vi "WPI_MotorControlGetOutput.vi"(8 "error in":errorcluster, 11 "MotorControlDevRef":T1={"DeviceStatus"={"status"=FALSE, "code"=0, "source"=""}, "Type"=enum."PWM", "PWM"={"PWM Channel"=enum."Invalid", "DeadBand"={"Name"="", "maxPositivePwm"=0, "minPositivePwm"=0, "centerPwm"=0, "maxNegativePwm"=0, "minNegativePwm"=0, "angularRange"=0}}, "CAN"={"Device Number"=0, "SetOutput VI Ref"=variant(refnum<vi> refnum), "GetOutput VI Ref"=variant(refnum<vi> refnum), "Enable VI Ref"=variant(refnum<vi> refnum), "Disable VI Ref"=variant(refnum<vi> refnum), "Data"=variant}, "Invert"=FALSE, "DIO PWM"={"PWM \"Enable\" Channel"=enum."Invalid", "DIOChannel"=enum."Invalid", "PWM Rate"=0.0}}) -> (0 "error out":errorcluster, 2 "Output":dbl, 3 "MotorControlDevRef":T1={"DeviceStatus"={"status"=FALSE, "code"=0, "source"=""}, "Type"=enum."PWM", "PWM"={"PWM Channel"=enum."Invalid", "DeadBand"={"Name"="", "maxPositivePwm"=0, "minPositivePwm"=0, "centerPwm"=0, "maxNegativePwm"=0, "minNegativePwm"=0, "angularRange"=0}}, "CAN"={"Device Number"=0, "SetOutput VI Ref"=variant(refnum<vi> refnum), "GetOutput VI Ref"=variant(refnum<vi> refnum), "Enable VI Ref"=variant(refnum<vi> refnum), "Disable VI Ref"=variant(refnum<vi> refnum), "Data"=variant}, "Invert"=FALSE, "DIO PWM"={"PWM \"Enable\" Channel"=enum."Invalid", "DIOChannel"=enum."Invalid", "PWM Rate"=0.0}})   [LabVIEW 2025]
doc: "Returns the last output value or set-point that was written to the motor controller with the <B>Set Output</B> VI."
uses:
  <vilib>/Rock Robotics/WPI/MotorControl/WPI_MotorControlDeviceRef.ctl
  <vilib>/Rock Robotics/WPI/MotorControl/WPI_MotorControlType.ctl
  <vilib>/Rock Robotics/SystemInterfaces/DIO/FPGA_DIOPWMChannel.ctl
  <vilib>/Rock Robotics/WPI/PWM/WPI_PWMDeadband.ctl
  <vilib>/Rock Robotics/SystemInterfaces/DIO/FPGA_DIOChannel.ctl
  <vilib>/Rock Robotics/WPI/PWM/WPI_PWMChannelCacheOp.ctl
  <vilib>/Rock Robotics/WPI/MotorControl/WPI_MotorControlGetOutputRefType.ctl
  <vilib>/Rock Robotics/WPI/DigitalOutput/WPI_DigitalOutputDevRef.ctl
  <vilib>/Rock Robotics/WPI/Simulation/Protocol/Devices/PWM/PWM Update Ops.ctl
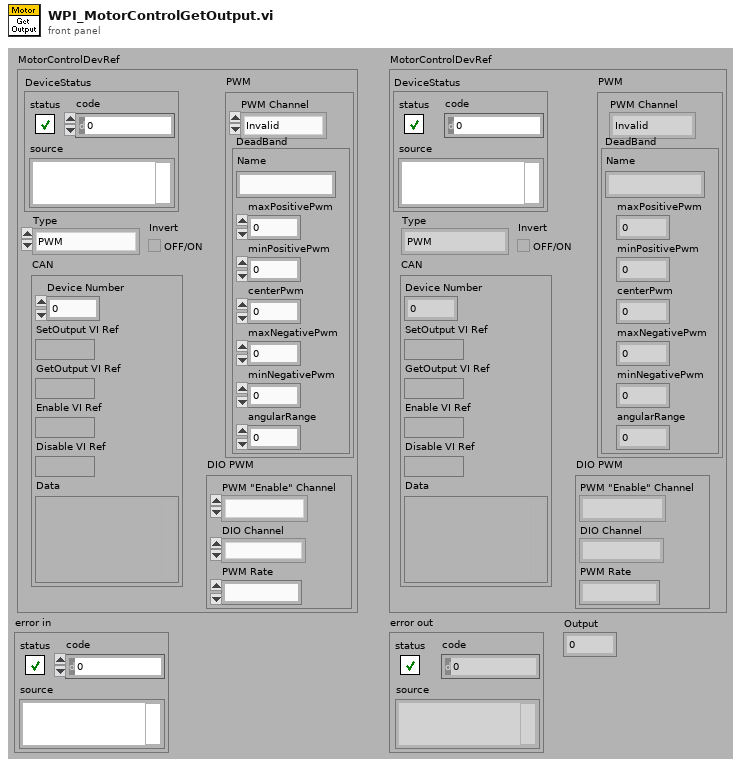
[diagram p1: front panel]
types:
  T1 = typedef "WPI_MotorControlDeviceRef.ctl" = cluster{"DeviceStatus":errorcluster, "Type":T2, "PWM":cluster{"PWM Channel":T3, "DeadBand":T4}, "CAN":cluster{"Device Number":u8, "SetOutput VI Ref":variant, "GetOutput VI Ref":variant, "Enable VI Ref":variant, "Disable VI Ref":variant, "Data":variant}, "Invert":bool, "DIO PWM":cluster{"PWM \"Enable\" Channel":T3, "DIOChannel":T5, "PWM Rate":dbl}}
  T2 = typedef "WPI_MotorControlType.ctl" = enum16{"PWM", "CAN", "DIO PWM"}
  T3 = typedef "FPGA_DIOPWMChannel.ctl" = enum8{"PWM 0", "PWM 1", "PWM 2", "PWM 3", "PWM 4", "PWM 5", "PWM 6", "PWM 7", "PWM 8", "PWM 9", "PWM MXP 0", "PWM MXP 1", "PWM MXP 2", "PWM MXP 3", "PWM MXP 4", "PWM MXP 5", "PWM MXP 6", "PWM MXP 7", "PWM MXP 8", "PWM MXP 9", "Invalid"}
  T4 = typedef "WPI_PWMDeadband.ctl" = cluster{"Name":string, "maxPositivePwm":i32, "minPositivePwm":i32, "centerPwm":i32, "maxNegativePwm":i32, "minNegativePwm":i32, "angularRange":u16}
  T5 = typedef "FPGA_DIOChannel.ctl" = enum8{"DIO 0", "DIO 1", "DIO 2", "DIO 3", "DIO 4", "DIO 5", "DIO 6", "DIO 7", "DIO 8", "DIO 9", "DIO MXP 0", "DIO MXP 1", "DIO MXP 2", "DIO MXP 3", "DIO MXP 4", "DIO MXP 5", "DIO MXP 6", "DIO MXP 7", "DIO MXP 8", "DIO MXP 9", "DIO MXP 10", "DIO MXP 11", "DIO MXP 12", "DIO MXP 13", "DIO MXP 14", "DIO MXP 15", "SPI Port CS1", "SPI Port CS2", "SPI Port CS3", "SPI Port MISO", "SPI Port MOSI", "Invalid"}
  T6 = typedef "WPI_MotorControlGetOutputRefType.ctl" = refnum<vi>
  T7 = typedef "WPI_DigitalOutputDevRef.ctl" = cluster{"DIO Channel":T5, "DevStatus":errorcluster}
  T8 = typedef "PWM Update Ops.ctl" = enum16{"set init", "set speed", "set position", "set raw", "set  period_scale", "set zero_latch", "set angular range", "get", "delete", "JSON update", "set name", "transmit initial", "reset"}
  T9 = typedef "WPI_PWMChannelCacheOp.ctl" = enum16{"Acquire", "Release", "Status"}
  T10 = typedef "WPI_PWMDeviceRef.ctl" = cluster{"DeviceStatus":errorcluster, "PWM Channel":T3}
  T11 = typedef "PWM proto.ctl" = cluster{"type":string, "device":string, "name":string, "data":T12}
  T12 = typedef "PWM data proto.ctl" = cluster{"<init":bool, "<speed":dbl, "<position":dbl, "<raw":dbl, "<period_scale":dbl, "<zero_latch":bool, "<servo range":dbl}
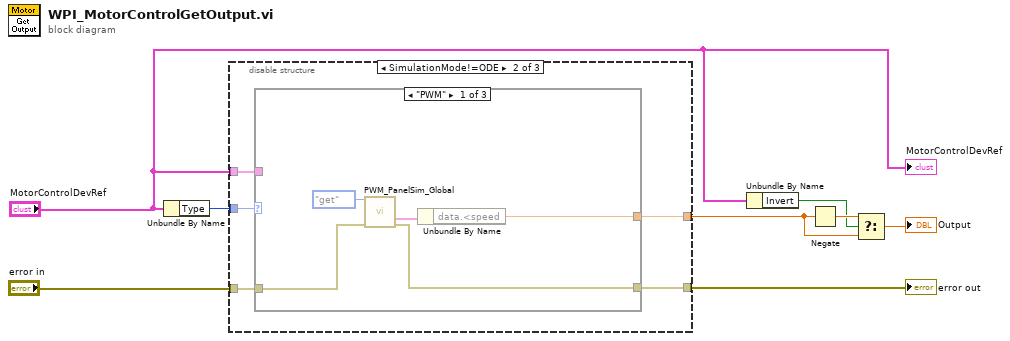
[diagram p0: block diagram]
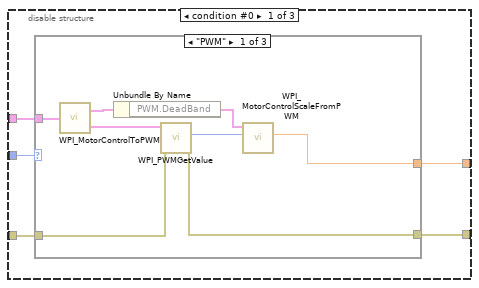
[diagram p2: hidden frame]
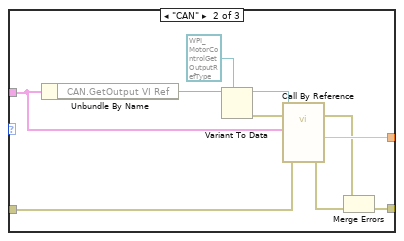
[diagram p3: hidden frame]
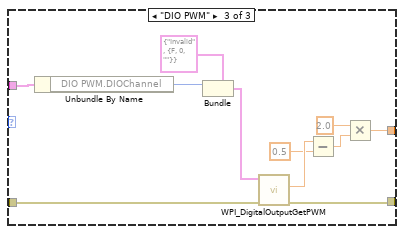
[diagram p4: hidden frame]
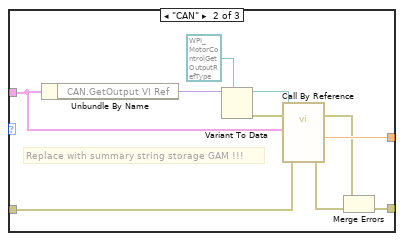
[diagram p5: hidden frame]
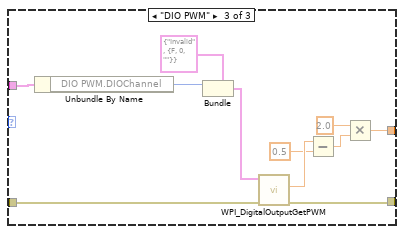
[diagram p6: hidden frame]
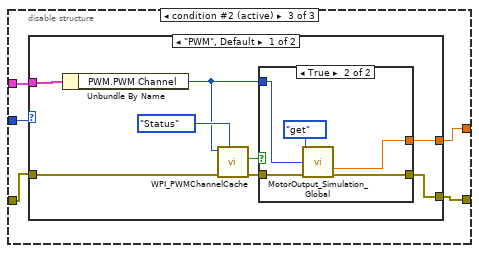
[diagram p7: hidden frame]
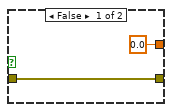
[diagram p8: hidden frame]
diagram:
  n1 = Unbundle By Name("MotorControlDevRef") -> ("Type"=w2:T2)
  n2 = disable-structure shown="SimulationMode!=ODE" {
    disable-tunnel: "error in" -> [w13 w45 w76]
    disable-tunnel: "MotorControlDevRef" -> [w12 w43 w78]
    disable-tunnel: [w11 w47 w74] -> w6
    disable-tunnel: w2 -> [w10 w44 w77]
    disable-tunnel: [w9 w46 w75] -> w1
    frame condition #0 {
      n3 = case shown="\"PWM\"" w10 {
        tunnel: [w14 w23 w37] -> w11
        tunnel: w12 -> [w17 w27 w42]
        tunnel: w13 -> [w15 w29 w38]
        tunnel: [w20 w30 w33] -> w9
        frame "PWM" {
          n4 = call <vilib>:"WPI_MotorControlToPWM.vi"("MotorControlDeviceRef"=w17) -> ("MotorControlDeviceRef"=w16:T1, "PWMDeviceRef"=w19:T10)
          n5 = Unbundle By Name(w16) -> ("PWM.DeadBand"=w18:T4)
          n6 = call <vilib>:"WPI_PWMGetValue.vi"("error in (no error)"=w15, "PWMDeviceRef"=w19) -> ("error out"=w14:errorcluster, "Value"=w21:u16)  [unwired: 8 out]
          n7 = call <vilib>:"WPI_MotorControlScaleFromPWM.vi"("Raw PWM Value"=w21, "DeadBand Info"=w18) -> ("Output (1,-1)"=w20:dbl)  [unwired: 9 out]
        }
        frame "CAN" {
          n8 = Unbundle By Name(w27) -> ("CAN.GetOutput VI Ref"=w31:variant)
          n9 = Variant To Data(type=T6 refnum ("MotorControlGetOutput"), Variant=w31) -> (data=w28:T6, error out=w26:errorcluster)  [unwired: 1 in]
          n10 = call-by-ref "?"(reference=w28, error in=w26, "error in"=w29, "MotorControlDevRef"=w27) -> (error out=w25:errorcluster, 0:"error out"=w24:errorcluster, "Output"=w30:dbl)  [unwired: 7 in, 2 out]
          n11 = Merge Errors(w25, w24) -> (w23:errorcluster)
        }
        frame "DIO PWM" {
          n12 = Unbundle By Name(w42) -> ("DIO PWM.DIOChannel"=w40:T5)
          n13 = Bundle(cluster=T7 {"DIO Channel"=enum."Invalid", "DevStatus"={"status"=FALSE, "code"=0, "source"=""}} ("DigitalOutputDevRef"), "DIO Channel"=w40) -> (w39:T7)  [unwired: 1 in]
          n14 = call <vilib>:"WPI_DigitalOutputGetPWM.vi"("error in (no error)"=w38, "DigitalOutputDevRef"=w39) -> ("error out"=w37:errorcluster, "PWM Duty Cycle"=w36:sgl)  [unwired: 7 in, 1 out]
          n15 = Subtract(x=w36, y=sgl 0.5) -> (x-y=w34:sgl)
          n16 = Multiply(x=sgl 2.0, y=w34) -> (x*y=w33:sgl)
        }
      }
    }
    frame condition #1 {
      n17 = case shown="\"PWM\"" w44 {
        tunnel: [w49 w54 w68] -> w47
        tunnel: w43 -> [_ w58 w73]
        tunnel: w45 -> [w48 w60 w69]
        tunnel: [w52 w61 w64] -> w46
        frame "PWM" {
          n18 = call <vilib>:"PWM_PanelSim_Global.vi"("menu"=PWM_Update_Ops."get", "error in (no error)"=w48) -> ("Value get"=w50:T11, "error out"=w49:errorcluster)  [unwired: 12 in]
          n19 = Unbundle By Name(w50) -> ("data.<speed"=w52:dbl)
        }
        frame "CAN" {
          # "Replace with summary string storage GAM !!!"
          n20 = Unbundle By Name(w58) -> ("CAN.GetOutput VI Ref"=w62:variant)
          n21 = Variant To Data(type=T6 refnum ("MotorControlGetOutput"), Variant=w62) -> (data=w59:T6, error out=w57:errorcluster)  [unwired: 1 in]
          n22 = call-by-ref "?"(reference=w59, error in=w57, "error in"=w60, "MotorControlDevRef"=w58) -> (error out=w56:errorcluster, 0:"error out"=w55:errorcluster, "Output"=w61:dbl)  [unwired: 7 in, 2 out]
          n23 = Merge Errors(w56, w55) -> (w54:errorcluster)
        }
        frame "DIO PWM" {
          n24 = Unbundle By Name(w73) -> ("DIO PWM.DIOChannel"=w71:T5)
          n25 = Bundle(cluster=T7 {"DIO Channel"=enum."Invalid", "DevStatus"={"status"=FALSE, "code"=0, "source"=""}} ("DigitalOutputDevRef"), "DIO Channel"=w71) -> (w70:T7)  [unwired: 1 in]
          n26 = call <vilib>:"WPI_DigitalOutputGetPWM.vi"("error in (no error)"=w69, "DigitalOutputDevRef"=w70) -> ("error out"=w68:errorcluster, "PWM Duty Cycle"=w67:sgl)  [unwired: 7 in, 1 out]
          n27 = Subtract(x=w67, y=sgl 0.5) -> (x-y=w65:sgl)
          n28 = Multiply(x=sgl 2.0, y=w65) -> (x*y=w64:sgl)
        }
      }
    }
    frame condition #2 (active) {
      n29 = case shown="\"PWM\", Default" w77 {
        tunnel: [w79 w94] -> w74
        tunnel: [w80 _] -> w75
        tunnel: w78 -> [w86 _]
        tunnel: w76 -> [w84 w94]
        frame "PWM", Default {
          n30 = Unbundle By Name(w86) -> ("PWM.PWM Channel"=w81:T3)
          n31 = call <vilib>:"WPI_PWMChannelCache.vi"("Operation"=WPI_PWMChannelCacheOp."Status", "error in (no error)"=w84, "PWMChannel"=w81) -> ("error out"=w82:errorcluster, "Allocated?"=w83:bool)  [unwired: 2 in, 5 out]
          n32 = case shown="True" w83 {
            tunnel: w82 -> [w87 w92]
            tunnel: w81 -> [_ w91]
            tunnel: [0.0 ("Output Get") w90] -> w80
            tunnel: [w87 w89] -> w79
            frame False {
            }
            frame True {
              n33 = call <vilib>:"MotorOutput_Simulation_Global.vi"("menu"=enum16{"set", "get", "delete"}."get", "PWM Channel"=w91, "error in (no error)"=w92) -> ("Output Get"=w90:dbl, "error out"=w89:errorcluster)  [unwired: 11 in]
            }
          }
        }
        frame "CAN" {
        }
      }
    }
  }
  "error out" <- w6
  n34 = Unbundle By Name("MotorControlDevRef") -> ("Invert"=w3:bool)
  n35 = Negate(x=w1) -> (-x=w5:dbl)
  n36 = Select(t=w5, s=w3, f=w1) -> (s? t:f=→"Output":dbl)
  "MotorControlDevRef" <- "MotorControlDevRef"
